vi "test Deploy Scripted System Definition.vi"(8 "error in (no error)":errorcluster, 11 "TestCase in":refnum<class "Engine Simulation Scripting API System Tests.lvclass">) -> (0 "error out":errorcluster, 3 "TestCase out":refnum<class "Engine Simulation Scripting API System Tests.lvclass">)   [LabVIEW 2019, in "Engine Simulation Scripting API System Tests.lvclass"]
uses:
  Engine Simulation Scripting API System Tests.lvclass
  <vilib>/addons/_JKI Toolkits/VI Tester/TestCase.llb/TestCase.lvclass
  Scripting API/Engine Simulation Toolkit Scripting API.lvlib
  Scripting API/Bitfile/Bitfile.ctl
  <vilib>/NI/VeriStand Custom Device Testing Tools/VeriStandTestUtilities/VeriStandTestUtilities.lvlib
  Scripting API/APU/APU Settings.ctl
  NationalInstruments.VeriStand.SystemDefinitionAPI
  <userlib>/_OpenG.lib/file/file.llb/Append Path to Root if Relative - Scalar__ogtk.vi
  C:/Program Files (x86)/National Instruments/LabVIEW 2019/vi.lib/addons/_JKI Toolkits/VI Tester/TestCase.llb/TestCase.lvclass
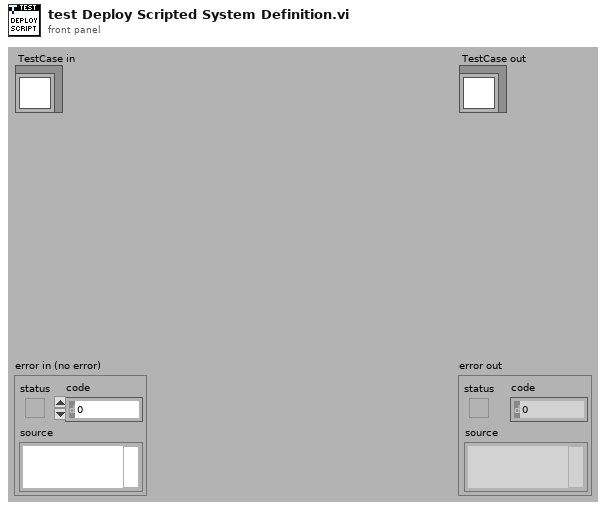
[diagram p1: front panel]
types:
  T1 = typedef "Engine Simulation Toolkit Scripting API.lvlib/APU Settings.ctl" = cluster{"Name":string, "Start angle (degrees)":dbl, "des speed":dbl, "Acceleration":bool, "des accel":dbl, "Maximum angle deviation\nbetween RIO devices (degrees)":dbl}
  T2 = typedef "Engine Simulation Toolkit Scripting API.lvlib/Bitfile.ctl" = cluster{"RIO Device Address":string, "Bitfile Path":path}
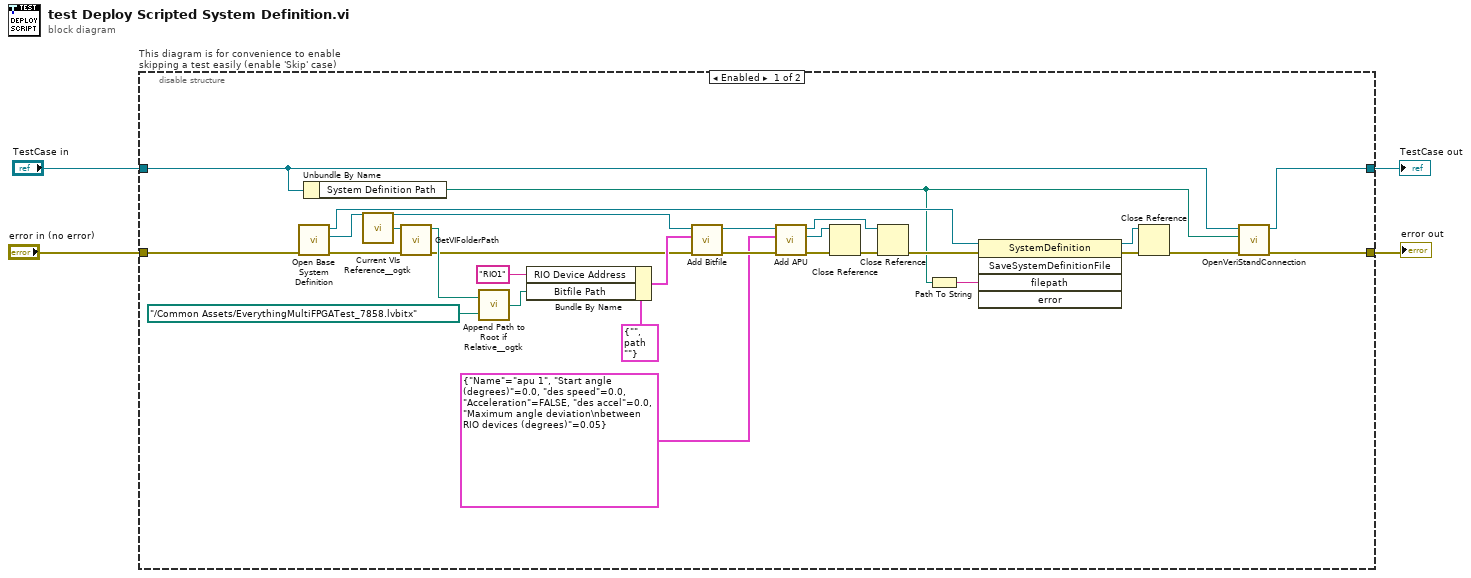
[diagram p0: block diagram]
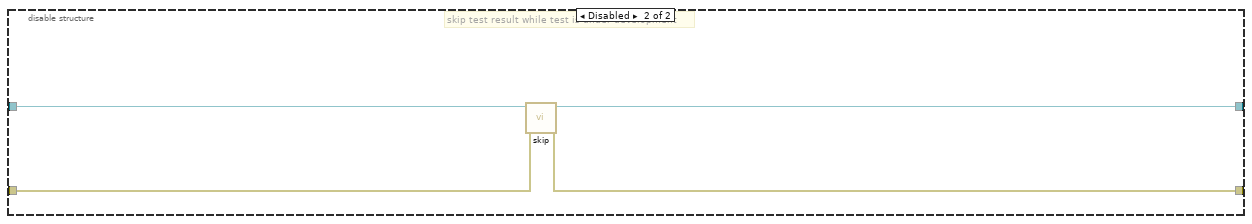
[diagram p2: hidden frame]
diagram:
  n1 = disable-structure "This diagram is for convenience to enable skipping a test easily (enable 'Skip' case)" shown="Enabled" {
    disable-tunnel: "TestCase in" -> [w30 w36]
    disable-tunnel: [w32 w34] -> w1
    disable-tunnel: [w31 w35] -> w3
    disable-tunnel: "error in (no error)" -> [w29 w33]
    frame Enabled {
      n2 = call "Open Base System Definition.vi"("error in (no error)"=w29) -> ("error out"=w24:errorcluster, "EST Custom Device"=w28:refnum<k24>, "SystemDefinition"=w11:refnum<k24>)  [unwired: 8 in]
      n3 = Unbundle By Name(w30) -> ("System Definition Path"=w6:path)
      n4 = call <userlib>:"Current VIs Reference__ogtk.vi"() -> ("Current VI's reference"=w27:refnum<vi>)  [unwired: 5 in]
      n5 = call <vilib>:"GetVIFolderPath.vi"("error in (no error)"=w24, "VI Reference in"=w27) -> ("error out"=w19:errorcluster, "VI Folder Path out"=w26:path)  [unwired: 8 in]
      n6 = call-poly <userlib>:"Append Path to Root if Relative__ogtk.vi"("Absolute or Relative Path"=path "../Common Assets/EverythingMultiFPGATest_7858.lvbitx", "Root Path"=w26) -> ("Absolute or Appended Path"=w21:path)
      n7 = Bundle By Name(cluster=T2 {"RIO Device Address"="", "Bitfile Path"=path ""} ("Engine Simulation Toolkit Bitfile"), "RIO Device Address"="RIO1", "Bitfile Path"=w21) -> (w20:T2)
      n8 = call "Add Bitfile.vi"("error in (no error)"=w19, "Engine Simulation Toolkit Bitfile"=w20, "EST Custom Device in"=w28) -> ("error out"=w17:errorcluster, "EST Custom Device out"=w18:refnum<k24>)  [unwired: 7 in]
      n9 = call "Add APU.vi"("error in (no error)"=w17, "APU Settings"=T1 {"Name"="apu 1", "Start angle (degrees)"=0.0, "des speed"=0.0, "Acceleration"=FALSE, "des accel"=0.0, "Maximum angle deviation\nbetween RIO devices (degrees)"=0.05}, "EST Custom Device in"=w18) -> ("error out"=w15:errorcluster, "APU"=w14:refnum<k24>, "EST Custom Device out"=w12:refnum<k24>)  [unwired: 6 in]
      n10 = Close Reference(reference=w14, error in (no error)=w15) -> (error out=w13:errorcluster)
      n11 = Close Reference(reference=w12, error in (no error)=w13) -> (error out=w7:errorcluster)
      n12 = Path To String(path=w6) -> (string=w8:string)
      n13 = invoke class="SystemDefinition" method="SaveSystemDefinitionFile"(reference=w11, error in=w7, "filepath"=w8) -> (reference out=w9:refnum<k24>, error out=w10:errorcluster)  [unwired: 2 in, 3 out]
      n14 = Close Reference(reference=w9, error in (no error)=w10) -> (error out=w5:errorcluster)
      n15 = call-dynamic "OpenVeriStandConnection.vi"("error in (no error)"=w5, "System Definition File"=w6, "VeriStand Test Case in"=w30) -> ("error out"=w31:errorcluster, "VeriStand Test Case out"=w32:refnum<class "Engine Simulation Scripting API System Tests.lvclass">)  [unwired: 6 in, 1 out]
    }
    frame Disabled {
      # "skip test result while test is under development"
      n16 = call <vilib>:"skip.vi"("error in (no error)"=w33, "TestCase in"=w36) -> ("error out"=w35:errorcluster, "TestCase out"=w34:refnum<class "Engine Simulation Scripting API System Tests.lvclass">)  [unwired: 8 in]
    }
  }
  "error out" <- w3
  "TestCase out" <- w1
